vi "Memory.Pointer.Read.Safe.1D.Bool.vi"(7 "count (-1: all)":i64=-1 format="%d elements", 8 "error in (no error)":errorcluster, 9 "offset (0)":u64 format="%d bytes", 10 "buffer in":bool[](array[boolean]), 11 "pointer in":refnum<class "Memory.Pointer.lvclass">) -> (0 "error out":errorcluster, 1 "offset out":u64 format="%d bytes", 2 "buffer out":bool[](array[boolean]), 3 "pointer out":refnum<class "Memory.Pointer.lvclass">)   [LabVIEW 2016, in "Memory.lvlib" / "Memory.Pointer.lvclass"]
doc: "Reads <b>count</b> elements from the address specified by <b>pointer + offset</b> into the provided <b>buffer</b>.\n\n<b>Note:</b> This VI is <b>safe</b>.\n\nSafe means that this function evaluates the size parameter of <b>pointer</b> to ensure that is inbounds of allocated memory before peforming a memory read/write. Reading/writing more data to a pointer than it has allocated can corrupt or crash LabVIEW."
uses:
  Memory.Pointer.lvclass
  Memory.Pointer.lvclass/Memory.Pointer.ctl
  Memory.Pointer.Get Address.vi
  Memory.Pointer.Errors.vi
  Memory.Pointer.Errors.Null Pointer.vi
  Memory.Pointer.Errors.Out of Bounds.vi
  Memory.Pointer.Get Size.vi
  VIs/Memory.Count to Size.Power of 2.vi
  Memory.Pointer.Errors.Create Error.vi
  Submodules/SEH/Source/VIs/Static Error Handling.Source Buffer.Write.String.vi
  Memory.Pointer.Errors.Write Pointer Size.vi
  Submodules/SEH/Source/VIs/Static Error Handling.Source Buffer.Write.Numeric.Scalar.Base10.vi
  Submodules/SEH/Source/VIs/Static Error Handling.Source Buffer.Write.Numeric.Scalar.Base10 (U64).vi
  Submodules/SEH/Source/VIs/Static Error Handling.Error Cluster Constant.vi
  Submodules/SEH/Source/VIs/Static Error Handling.Error Cluster Constant (256B).vi
  Submodules/SEH/Source/VIs/Static Error Handling.Parameters.Status.Set.vi
  Submodules/SEH/Source/VIs/Static Error Handling.Parameters.Code.Set.vi
  Submodules/SEH/Source/VIs/Static Error Handling.Parameters.VI Source.Set.vi
  Constants/Memory.Constants.vi
  Constants/Memory.Constants.Library Name.vi
  Memory.Pointer.Errors.Get Info.vi
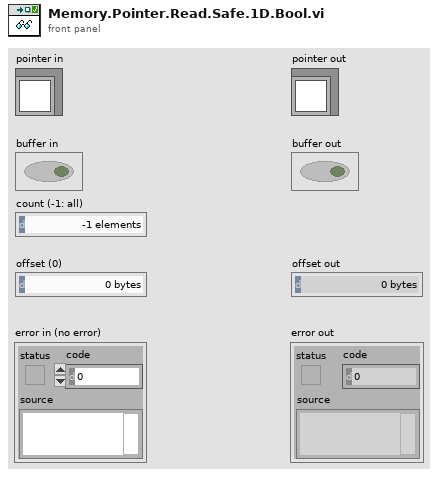
[diagram p1: front panel]
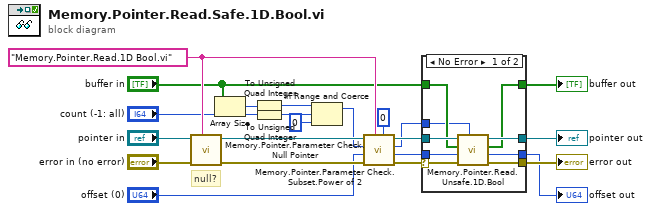
[diagram p0: block diagram]
diagram:
  w11 = "Memory.Pointer.Read.1D Bool.vi" ("source vi name")
  # "null?"
  n1 = call "Memory.Pointer.Parameter Check.Null Pointer.vi"("source vi name"=w11, "error in (no error)"="error in (no error)", "Pointer in"="pointer in") -> ("error out"=w12:errorcluster, "Pointer out"=w13:refnum<class "Memory.Pointer.lvclass">)  [unwired: 7 in]
  n2 = Array Size(array="buffer in") -> (size(s)=w10:i32)
  n3 = To Unsigned Quad Integer(1:w10) -> (0:w7:u64)
  n4 = To Unsigned Quad Integer(1:"count (-1: all)") -> (0:w8:u64)
  n5 = In Range and Coerce(upper limit=w7, x=w8, lower limit=u64 0) -> (coerced(x)=w6:u64)  [unwired: 1 out]
  n6 = call "Memory.Pointer.Parameter Check.Subset.Power of 2.vi"("power of 2"=i16 0, "source vi name"=w11, "error in (no error)"=w12, "offset (0)"="offset (0)", "count"=w6, "Pointer in"=w13) -> ("error out"=w22:errorcluster, "offset out"=w20:u64, "count"=w5:u64, "Pointer out"=w21:refnum<class "Memory.Pointer.lvclass">)  [unwired: 2 in]
  n7 = case shown="No Error" w22 {
    selector: w22 -> [w31 w34]
    tunnel: w21 -> [w29 w33]
    tunnel: w20 -> [w30 w35]
    tunnel: "buffer in" -> [w25 w32]
    tunnel: [w28 w34] -> w19
    tunnel: [w27 w33] -> w18
    tunnel: [w26 w35] -> w1
    tunnel: [w24 w32] -> w17
    tunnel: w5 -> [w23 _]
    frame No Error {
      n8 = call "Memory.Pointer.Read.Unsafe.1D.Bool.vi"("count"=w23, "error in (no error)"=w31, "offset (0)"=w30, "buffer in"=w25, "pointer in"=w29) -> ("error out"=w28:errorcluster, "offset out"=w26:u64, "buffer out"=w24:bool[], "pointer out"=w27:refnum<class "Memory.Pointer.lvclass">)  [unwired: 3 in]
    }
    frame Error {
    }
  }
  "error out" <- w19
  "pointer out" <- w18
  "buffer out" <- w17
  "offset out" <- w1
